vi "ExposeUpdateParameter.vi"(8 "error in (no error)":errorcluster, 9 "Name (empty)":string, 10 "Parameter":variant, 11 "Expose Info":T1) -> (0 "error out":errorcluster)   [LabVIEW 2017]
uses:
  Core/ExposeInfo.ctl
  C:/Code/CMCryoSysCode/Expose/COM/CSCom/CSCom/bin/Release/CSCom.dll
  COM/CSCom/CSCom/bin/Release/CSCom.dll
  Core/ExposeMessage.ctl
  Events/ExposeMessageType.ctl
  Mapper/ExposeObjectMapNamepathData.ctl
  Mapper/ExposeMapperDataTypeEnum.ctl
  Mapper/ExposeObjectMapContainerTypeEnum.ctl
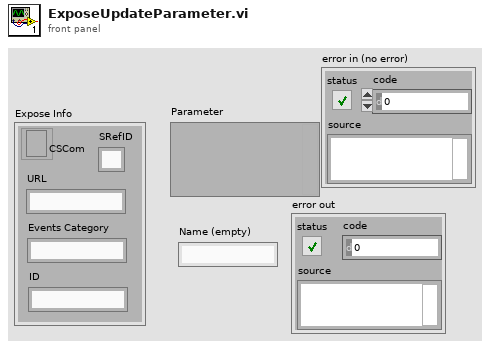
[diagram p1: front panel]
types:
  T1 = typedef "ExposeInfo.ctl" = cluster{"CSCom":refnum<k24>, "URL":string, "Events Category":string, "ID":string, "SRefID":string}
  T2 = typedef "ExposeMessage.ctl" = cluster{"Message Type":T3, "Text":string, "NamepathInfo":T4[]}
  T3 = typedef "ExposeMessageType.ctl" = i32
  T4 = typedef "ExposeObjectMapNamepathData.ctl" = cluster{"Type":T5, "Value":variant, "Namepath":string, "Container Type":T6}
  T5 = typedef "ExposeMapperDataTypeEnum.ctl" = enum16{"NotData", "int8", "byte", "int16", "uint16", "int32", "uint32", "int64", "uint64", "Single", "Double", "String", "Boolean", "Container"}
  T6 = typedef "ExposeObjectMapContainerTypeEnum.ctl" = enum16{"Value", "Array", "Waveform", "NetContainer"}
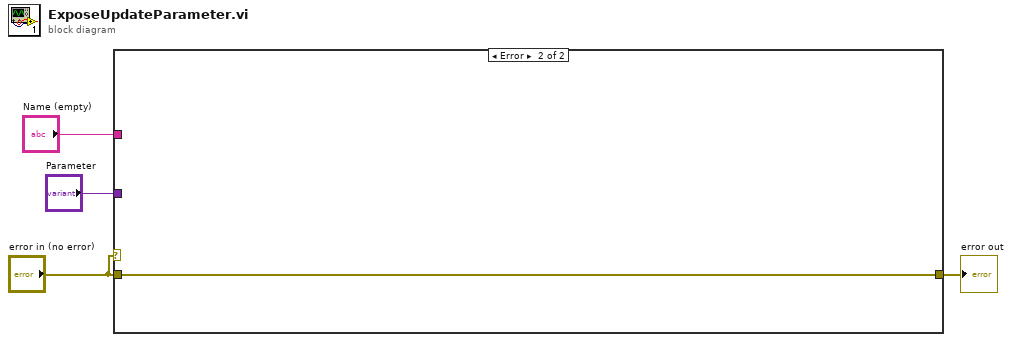
[diagram p0: block diagram]
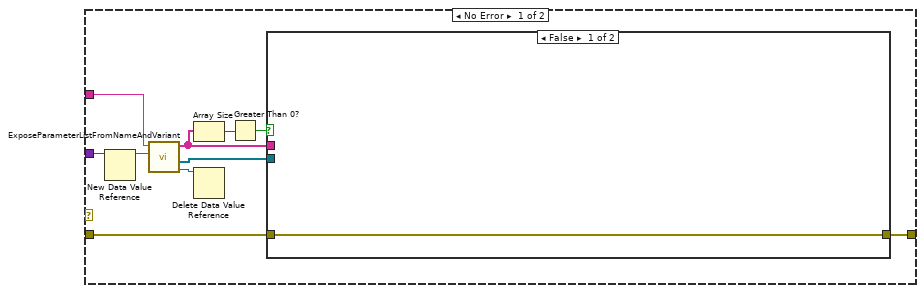
[diagram p2: hidden frame]
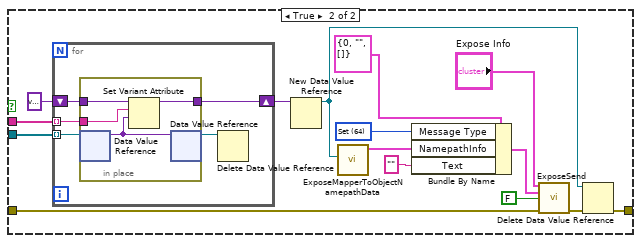
[diagram p3: hidden frame]
diagram:
  n1 = case shown="Error" "error in (no error)" {
    tunnel: "Name (empty)" -> [w14 _]
    tunnel: "Parameter" -> [w11 _]
    tunnel: "error in (no error)" -> [w6 w40]
    tunnel: [w5 w40] -> w2
    frame No Error {
      n2 = New Data Value Reference(data value=w11) -> (data value reference=w10:refnum<data-value>)  [unwired: 1 in, 1 out]
      n3 = call "ExposeParameterListFromNameAndVariant.vi"("Value Reference In"=w10, "Name (empty)"=w14) -> ("Value Reference Out"=w8:refnum<data-value>, "Parmaeter Refs"=w9:refnum<data-value>[], "Parameter names"=w7:string[])  [unwired: 7 in]
      n4 = Array Size(array=w7) -> (size(s)=w13:i32)
      n5 = Delete Data Value Reference(data value reference=w8) -> ()  [unwired: 1 in, 2 out]
      n6 = Greater Than 0?(x=w13) -> (x > 0?=w12:bool)
      n7 = case shown="False" w12 {
        tunnel: w7 -> [_ w29]
        tunnel: w9 -> [_ w21]
        tunnel: w6 -> [w15 w17]
        tunnel: [w15 w16] -> w5
        frame False {
        }
        frame True {
          w25 = T3 64 items=["Error"=1, "Warning"=2, "Create"=4, "Destroy"=8, "Invoke"=16, "Get"=32, "Set"=64, "Response"=128] ("Message Type")
          n8 = for {
            tunnel: w29 -> [w33] mode=indexing
            shift-right: [w34] -> w20
            shift-left: variant -> [w35]
            tunnel: w21 -> [w32] mode=indexing
            n9 = in-place {
              in-place-border: w35 -> [w39]
              in-place-border: [w38] -> w34
              in-place-border: w33 -> [w37]
              n10 = in-place-dvr #1(w32) -> (w36:variant)  [unwired: 1 out]
              n11 = Set Variant Attribute(Variant=w39, name=w37, value=w36) -> (Variant out=w38:variant)  [unwired: 1 in, 2 out]
              n12 = in-place-dvr #1(w36) -> (w31:refnum<data-value>)  [unwired: 1 out]
            }
            n13 = Delete Data Value Reference(data value reference=w31) -> ()  [unwired: 1 in, 2 out]
          }
          n14 = New Data Value Reference(data value=w20) -> (data value reference=w18:refnum<data-value>)  [unwired: 1 in, 1 out]
          n15 = call "ExposeMapperToObjectNamepathData.vi"("Value Reference In"=w18) -> ("Object map"=w22:T4[])  [unwired: 10 in]
          n16 = Bundle By Name(cluster=T2 {"Message Type"=0, "Text"="", "NamepathInfo"=[]} ("Message"), "Message Type"=w25, "NamepathInfo"=w22, "Text"="") -> (w27:T2)
          n17 = call "ExposeSend.vi"("Expose"="Expose Info", "Message"=w27, "Require Response"=FALSE, "error in (no error)"=w17) -> ("error out"=w19:errorcluster)  [unwired: 9 in, 2 out]
          n18 = Delete Data Value Reference(data value reference=w18, error in=w19) -> (error out=w16:errorcluster)  [unwired: 1 out]
        }
      }
    }
    frame Error {
    }
  }
  "error out" <- w2
